vi "Bottle_test_samples.vi"(10 "Pulse duration (ms)":dbl, 11 "Initial delay (ms)":dbl) -> (2 "leak samples start":i32, 3 "flow samples start":i32)   [LabVIEW 2016]
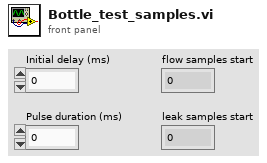
[diagram p1: front panel]
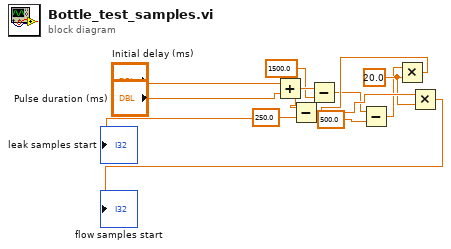
[diagram p0: block diagram]
diagram:
  w10 = 20.0 ("y")
  n1 = Add(x="Initial delay (ms)", y="Pulse duration (ms)") -> (x+y=w8:dbl)
  n2 = Subtract(x=w8, y=250.0) -> (x-y=w11:dbl)
  n3 = Subtract(x=w8, y=1500.0) -> (x-y=w3:dbl)
  n4 = Subtract(x=w3, y=500.0) -> (x-y=w5:dbl)
  n5 = Multiply(x=w5, y=w10) -> (x*y=→"leak samples start":dbl)
  n6 = Multiply(x=w11, y=w10) -> (x*y=→"flow samples start":dbl)
